vi "Modfiy_Local_Cost_Same_Values-1.vi"(3 "[IN] Cost Mutilplier":i8, 4 "[IN] Cost Function":i8[](array[numeric]), 5 "[IN] Array of Compared Values":dbl[](array[numeric])) -> (1 "[OUT] Cost Function":i8[](array[numeric]))   [LabVIEW 2013]
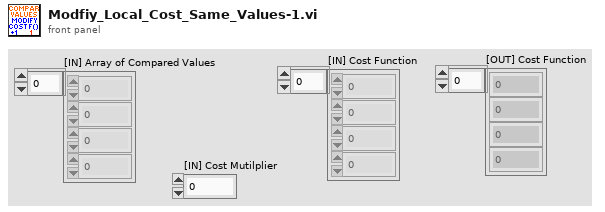
[diagram p1: front panel]
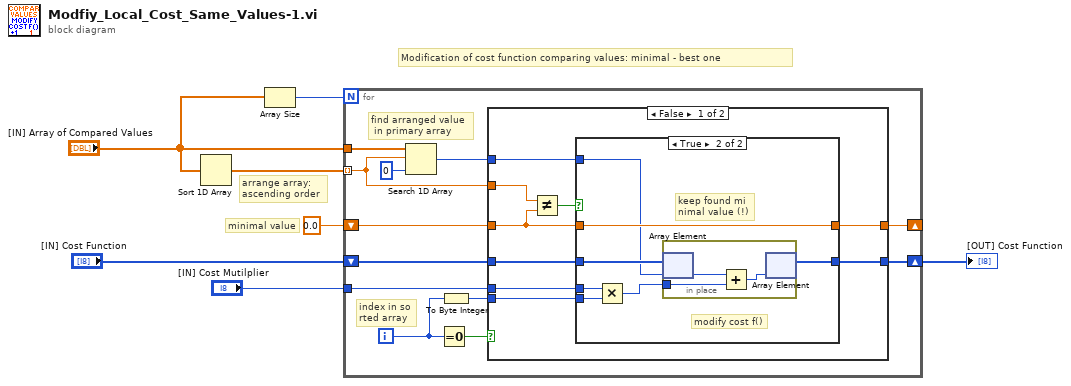
[diagram p0: block diagram]
diagram:
  # "minimal value"
  # "Modification of cost function comparing values: minimal - best one"
  # "arrange array: \nascending order"
  n1 = Sort 1D Array(array="[IN] Array of Compared Values") -> (sorted array=w7:dbl[])
  n2 = Array Size(array="[IN] Array of Compared Values") -> (size(s)=w1:i32)
  n3 = for {
    N: w1 -> [_]
    tunnel: w7 -> [w16] mode=indexing
    tunnel: "[IN] Array of Compared Values" -> [w19]
    shift-right: [w11] -> w3
    shift-left: "[IN] Cost Function" -> [w12]
    tunnel: "[IN] Cost Mutilplier" -> [w8]
    shift-right: [w15] -> _
    shift-left: 0.0 -> [w13]
    i -> [w10]
    # "find arranged value\n in primary array"
    # "index in so\nrted array"
    n4 = Search 1D Array(1D array=w19, element=w16, start index (0)=0) -> (index of element=w14:i32)
    n5 = Equal To 0?(x=w10) -> (x = 0?=w17:bool)
    n6 = To Byte Integer(number=w10) -> (8bit integer=w9:i8)
    n7 = case shown="False" w17 {
      tunnel: w16 -> [w27 w42]
      tunnel: [w26 w42] -> w15
      tunnel: w14 -> [w22 _]
      tunnel: w13 -> [w20 _]
      tunnel: w12 -> [w25 w41]
      tunnel: [w21 w41] -> w11
      tunnel: w9 -> [w24 _]
      tunnel: w8 -> [w23 _]
      frame False {
        n8 = Not Equal?(x=w27, y=w20) -> (x != y?=w28:bool)
        n9 = case shown="True" w28 {
          tunnel: w20 -> [w30 w37]
          tunnel: [w30 w37] -> w26
          tunnel: w25 -> [w29 w36]
          tunnel: w24 -> [_ w34]
          tunnel: w23 -> [_ w35]
          tunnel: w22 -> [_ w33]
          tunnel: [w29 w31] -> w21
          frame False {
            # "compared values are equal\n=> cost f() the same"
          }
          frame True {
            # "keep found mi\nnimal value (!)"
            # "modify cost f()"
            n10 = Multiply(x=w35, y=w34) -> (x*y=w32:i8)
            n11 = in-place {
              in-place-border: w32 -> [w39]
              n12 = in-place-array #1(w36, w33) -> (w40:i8)
              n13 = Add(x=w40, y=w39) -> (x+y=w38:i8)
              n14 = in-place-array #1(w38) -> (w31:i8[])  [unwired: 1 out]
            }
          }
        }
      }
      frame True {
        # "1st step: cost function isn't modified"
      }
    }
  }
  "[OUT] Cost Function" <- w3
